vi "Get Array Configuration.vi"(8 "error in (no error)":errorcluster, 11 "Core Threads Configuration in":refnum<class "Core Threads Configuration.lvclass">) -> (0 "error out":errorcluster, 2 "thread configurations":T1[](array[typedef]), 3 "Core Threads Configuration out":refnum<class "Core Threads Configuration.lvclass">)   [LabVIEW 2017, in "DSF Core.lvlib" / "Core Threads Configuration.lvclass"]
uses:
  Core Threads Configuration.lvclass
  Typedefs/DSF Core Thread Configuration.ctl
  Core Threads Configuration.lvclass/Core Threads Configuration.ctl
  DSF Core.lvlib
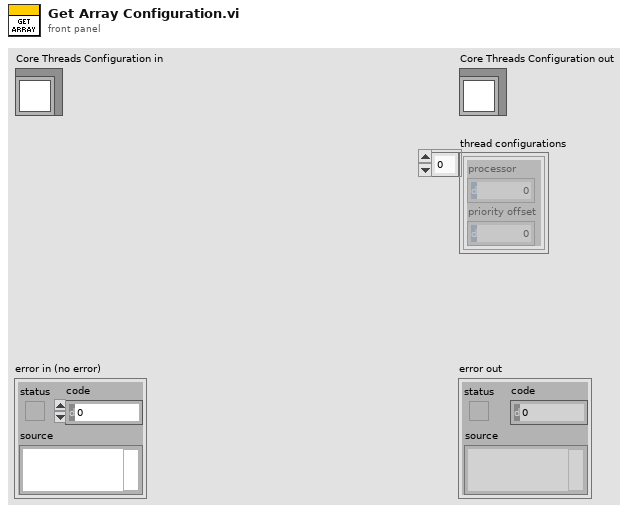
[diagram p1: front panel]
types:
  T1 = typedef "DSF Core.lvlib/DSF Core Thread Configuration.ctl" = cluster{"processor":i32, "priority offset":i16}
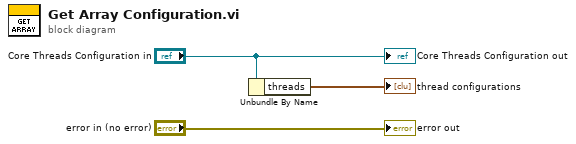
[diagram p0: block diagram]
diagram:
  n1 = Unbundle By Name("Core Threads Configuration in") -> ("threads"=→"thread configurations":T1[])
  "error out" <- "error in (no error)"
  "Core Threads Configuration out" <- "Core Threads Configuration in"
